vi "GetObject.vi"(4 "RefNum":i32, 5 "error in (no error)":errorcluster) -> (18 "reference":refnum<class "AbstractNode.lvclass">, 19 "error out":errorcluster)   [LabVIEW 2014, in "AbstractNode.lvclass"]
doc: "public Object clone()"
uses:
  <resource>/Framework/Providers/Open_GDS/UML/AbstractNode_class/AbstractNode.lvclass
  <resource>/Framework/Providers/Open_GDS/UML/AbstractNode_class/AbstractNode.lvclass/AbstractNode.ctl
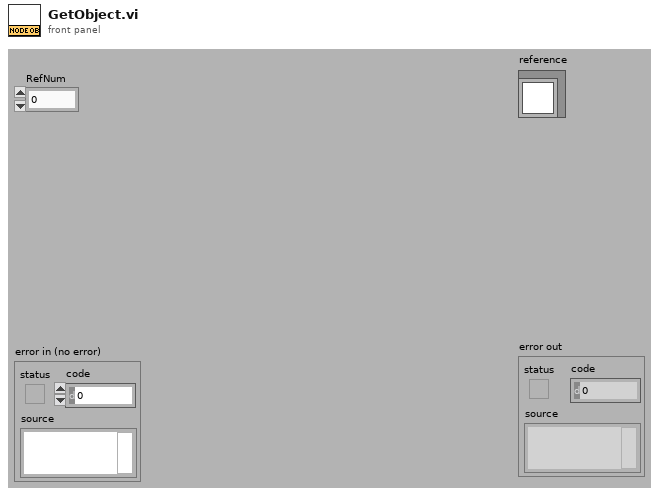
[diagram p1: front panel]
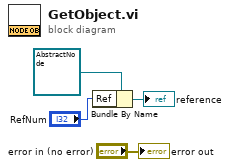
[diagram p0: block diagram]
diagram:
  n1 = Bundle By Name(cluster=refnum<class "AbstractNode.lvclass"> refnum ("reference"), "Ref"="RefNum") -> (→"reference":refnum<class "AbstractNode.lvclass">)
  "error out" <- "error in (no error)"
